vi "Dynamic call-Sys Config window.vi"(7 "Set tab page? (F)":bool, 8 "error in (no error)":errorcluster, 10 "System Config Tab Control":T1) -> (0 "error out":errorcluster)   [LabVIEW 2017]
uses:
  Windows/System config window/Typedefs/HW Setup tab control.ctl
  Windows/System config window/Globals/Sys Config window globals.vi
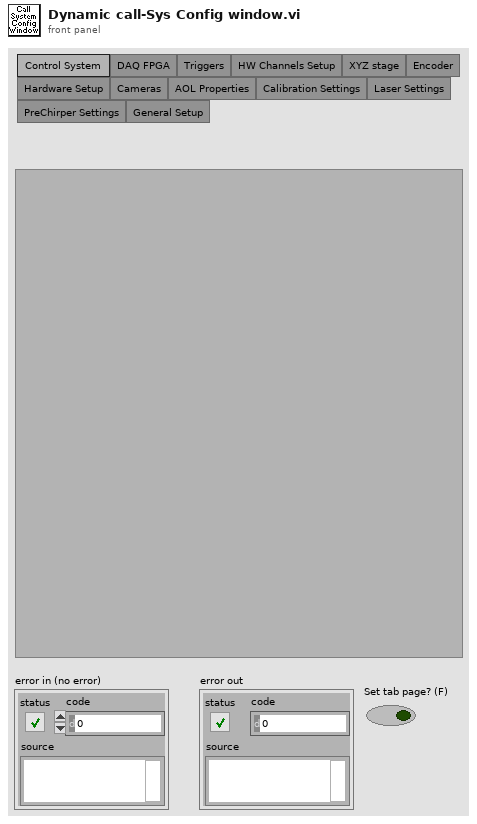
[diagram p1: front panel]
types:
  T1 = typedef "HW Setup tab control.ctl" = enum32{"Control System ", "DAQ FPGA", "Triggers", "HW Channels Setup", "XYZ stage", "Encoder", "Hardware Setup", "Cameras", "AOL Properties", "Calibration Settings", "Laser Settings", "PreChirper Settings", "General Setup"}
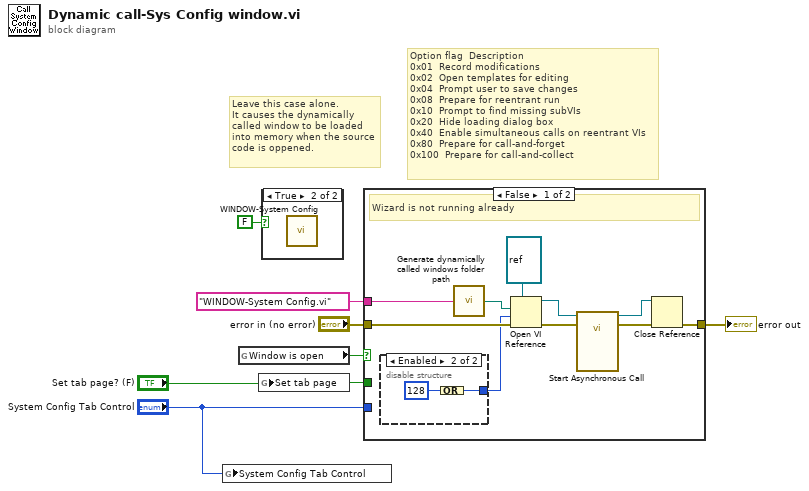
[diagram p0: block diagram]
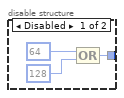
[diagram p3: hidden frame]
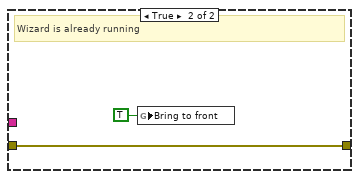
[diagram p4: hidden frame]
diagram:
  # "Leave this case alone.\nIt causes the dynamically called window to be loaded into memory when the source code is oppened."
  # "Option flag \tDescription\n0x01 \tRecord modifications\n0x02 \tOpen templates for editing\n0x04 \tPrompt user to save changes\n0x08 \tPrepare for reentrant run\n0x10 \tPrompt to find missing subVIs\n0x20 \tHide loading dialog box\n0x40 \tEnable simultaneous calls on reentrant VIs\n0x80 \tPrepare for call-and-forget\n0x100 \tPrepare for call-and-collect"
  n1 = global write "Sys Config window globals.vi" "System Config Tab Control"("System Config Tab Control") -> ()
  n2 = global read "Sys Config window globals.vi" "Window is open"() -> (w3:bool)
  n3 = global write "Sys Config window globals.vi" "Set tab page"("Set tab page? (F)") -> ()
  n4 = case shown="True" FALSE {
    frame False {
    }
    frame True {
      n5 = call "WINDOW-System Config.vi"() -> ()  [unwired: 12 in]
    }
  }
  n6 = case shown="False" w3 {
    tunnel: "error in (no error)" -> [w17 w24]
    tunnel: [w16 w24] -> w7
    tunnel: "WINDOW-System Config.vi" ("Error Source") -> [w14 _]
    tunnel: "Set tab page? (F)" -> [_ _]
    tunnel: "System Config Tab Control" -> [_ _]
    frame False {
      # "Wizard is not running already"
      n7 = disable-structure shown="Enabled" {
        disable-tunnel: [w20 w22] -> w11
        frame Disabled {
          n8 = Compound Arithmetic op=OR(64, 128) -> (w20:i32)
        }
        frame Enabled {
          n9 = Compound Arithmetic op=OR(128) -> (w22:i32)
        }
      }
      n10 = call "Generate dynamically called windows folder path.vi"("name of dynamically called VI"=w14) -> ("Dynamically called VI path"=w15:path)
      n11 = Open VI Reference(type specifier VI Refnum (for type only)=refnum<vi> refnum, vi path=w15, options=w11, error in (no error)=w17) -> (vi reference=w12:refnum<vi>, error out=w13:errorcluster)  [unwired: 2 in]
      n12 = call-by-ref "Start Asynchronous Call"(reference=w12, error in=w13) -> (reference out=w8:refnum<vi>, error out=w9:errorcluster)  [unwired: 12 in]
      n13 = Close Reference(reference=w8, error in (no error)=w9) -> (error out=w16:errorcluster)
    }
    frame True {
      # "Wizard is already running"
      n14 = global write "Sys Config window globals.vi" "Bring to front"(TRUE ("Bring to front")) -> ()
    }
  }
  "error out" <- w7
